vi "Remote_Request_Unit_Test.vi"() -> ()   [LabVIEW 2017]
uses:
  Controls/Packet/Packet.ctl
  Controls/Packet/Packet_Direction.ctl
  Controls/Packet/Packet_Type.ctl
  Controls/Packet/Packet_Priority.ctl
  Controls/Control Packets/RREQ_Param.ctl
panel:
  out "Raw Bytes":u8[][](array[numeric])
  out "Processed Bytes":u8[][](array[numeric])
  out "RREQ Param Out":T1
  out "RREQ Packet Out":T2
  in  "Retry interval (ms)":u32
  in  "Number of tries":u32
  in  "FIDs":u8[](array[numeric])
  in  "baud rate":u32=9600
  in  "COM Port In":refnum<visa-resource-name>
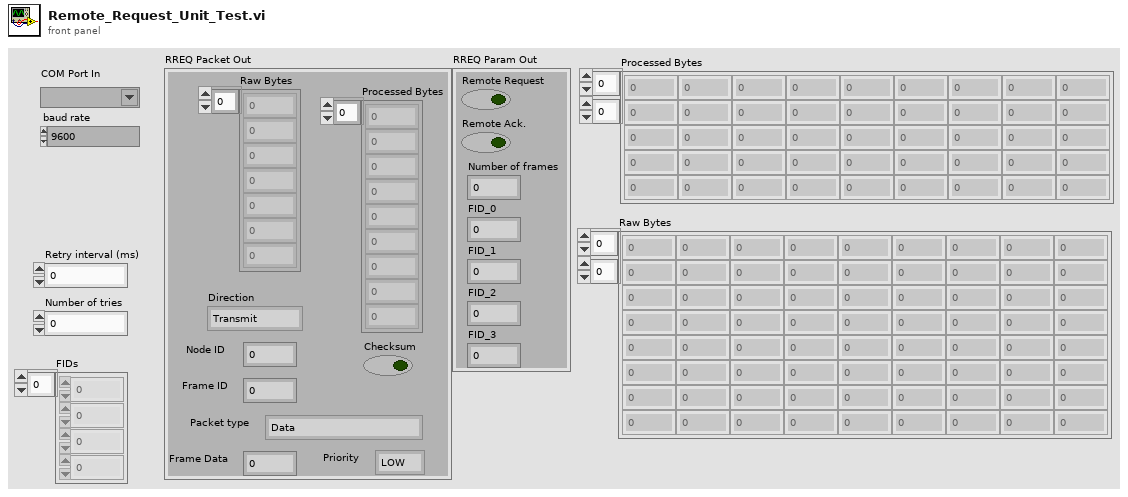
[diagram p1: front panel]
types:
  T1 = typedef "RREQ_Param.ctl" = cluster{"Remote Request":bool, "Remote Ack.":bool, "Number of frames":u8, "FID_0":u8, "FID_1":u8, "FID_2":u8, "FID_3":u8}
  T2 = typedef "Packet.ctl" = cluster{"Raw Bytes":u8[], "Checksum":bool, "Direction":T3, "Processed Bytes":u8[], "Node ID":u8, "Packet type":T4, "Frame Data":u32, "Priority":T5, "Frame ID":u8}
  T3 = typedef "Packet_Direction.ctl" = enum16{"Transmit", "Receive", "Bidirectional"}
  T4 = typedef "Packet_Type.ctl" = enum16{"Data", "Connection Management", "Remote Request", "Error/Status"}
  T5 = typedef "Packet_Priority.ctl" = enum16{"LOW", "HIGH"}
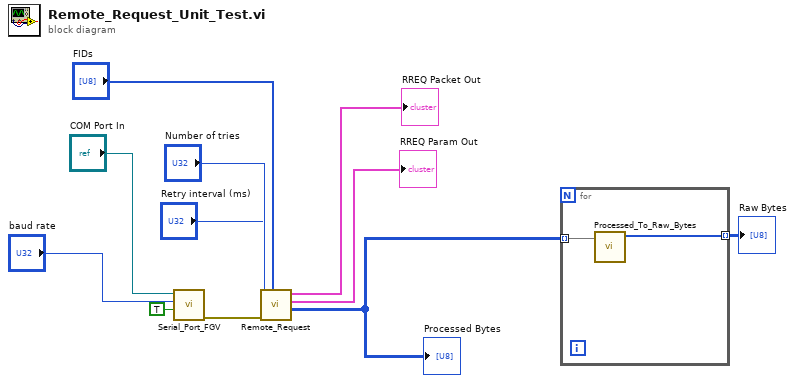
[diagram p0: block diagram]
diagram:
  n1 = call "Serial_Port_FGV.vi"("Initialize ?"=TRUE, "baud rate"="baud rate", "COM Port In"="COM Port In") -> ("error out"=w8:errorcluster)  [unwired: 7 in, 1 out]
  n2 = call "Remote_Request.vi"("FIDs"="FIDs", "error in (no error)"=w8, "Retry interval (ms)"="Retry interval (ms)", "Number of tries"="Number of tries") -> ("Processed Bytes"=w2:u8[][], "RREQ Param Out"=→"RREQ Param Out":T1, "RREQ Packet Out"=→"RREQ Packet Out":T2)  [unwired: 4 in, 1 out]
  "Processed Bytes" <- w2
  n3 = for {
    tunnel: w2 -> [w13] mode=indexing
    tunnel: [w12] -> w1 mode=indexing
    n4 = call "Processed_To_Raw_Bytes.vi"("Processed Bytes"=w13) -> ("Raw Bytes"=w12:u8[])  [unwired: 1 in, 4 out]
  }
  "Raw Bytes" <- w1
